vi "temp.vi"() -> ()   [LabVIEW 2012]
panel:
  in  "Stop Button":bool
  out "Characters Read":string
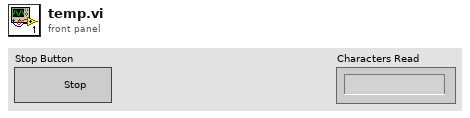
[diagram p1: front panel]
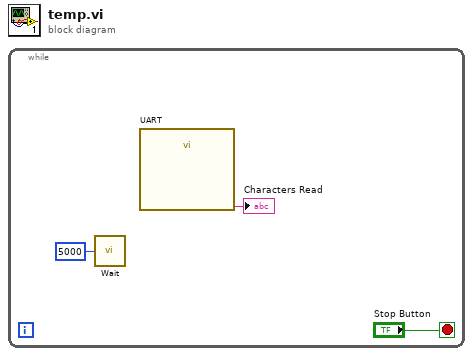
[diagram p0: block diagram]
diagram:
  n1 = while {
    stop <- "Stop Button" stop-if-true
    n2 = call "Wait"("Count(mSec)"=u32 5000) -> ()  [unwired: 1 out]
    n3 = call "UART"() -> ("Characters Read"=→"Characters Read":string)  [unwired: 26 in, 1 out]
  }
